vi "PID_to_Goal.vi"(8 "Boolean":bool, 10 "PID gains":T2, 11 "Direction to Goal":T1) -> (1 "Goal Arrive?":bool, 2 "PID Value":dbl, 3 "Frame Velocity":dbl[](array[numeric]))   [LabVIEW 2016]
uses:
  <vilib>/addons/control/pid/pid.llb/PID (DBL).vi
  <vilib>/addons/control/pid/NI_PID_pid.lvlib
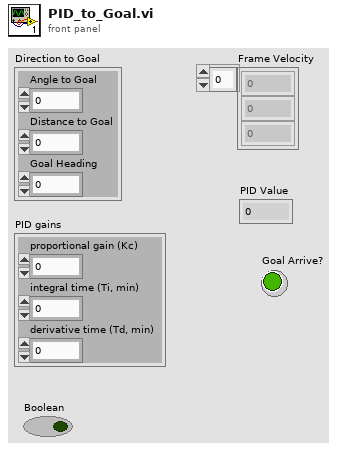
[diagram p1: front panel]
types:
  T1 = cluster{"Angle to Goal":dbl, "Distance to Goal":sgl, "Goal Heading":sgl}
  T2 = cluster{"proportional gain (Kc)":dbl, "integral time (Ti, min)":dbl, "derivative time (Td, min)":dbl}
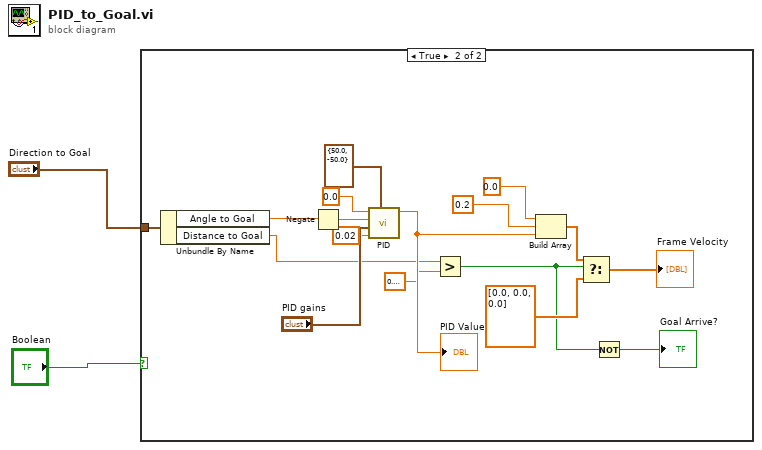
[diagram p0: block diagram]
diagram:
  n1 = case shown="True" "Boolean" {
    tunnel: "Direction to Goal" -> [_ w13]
    frame False {
    }
    frame True {
      n2 = Unbundle By Name(w13) -> ("Angle to Goal"=w14:dbl, "Distance to Goal"=w11:sgl)
      n3 = Negate(x=w14) -> (-x=w15:dbl)
      n4 = call-poly <vilib>:"PID.vi"("output range"=cluster{"output high":dbl, "output low":dbl} {"output high"=50.0, "output low"=-50.0}, "dt (s)"=0.02, "PID gains"="PID gains", "process variable"=w15, "setpoint"=0.0) -> ("output"=w18:dbl)  [unwired: 5 in, 1 out]
      "PID Value" <- w18
      n5 = Greater?(x=w11, y=sgl 0.3) -> (0:w5:bool)
      n6 = Build Array(0.0 ("element"), 0.2 ("element"), w18) -> (w8:dbl[])
      n7 = Select(t=w8, s=w5, f=dbl[] [0.0, 0.0, 0.0]) -> (s? t:f=→"Frame Velocity":dbl[])
      n8 = Not(x=w5) -> (.not. x?=→"Goal Arrive?":bool)
    }
  }
